vi "Teleop.vi"(10 "Match Info":T1={"Autonomous Elapsed Seconds"=0.0, "TeleOp Elapsed Seconds"=0.0, "Disabled Elapsed Seconds"=0.0, "Visited Autonomous"=FALSE, "Visited TeleOp"=FALSE, "Visited Disabled"=FALSE, "Autonomous Settings"={"Autonomous Style"=enum."Independent", "VI Refnum"=refnum}}, 11 "Call Context":T2) -> ()   [LabVIEW 2017]
doc: "This VI is called for each TeleOp packet received from the DS where the robot is not disabled. It is often used to read from the joysticks and update I/O or to update setpoints for timed control loops. It should complete and return within 20 milliseconds or it may miss DS packets."
uses:
  <vilib>/Rock Robotics/WPI/DriverStation/WPI_DriverStationDerivedRobotMode.ctl
  <vilib>/Rock Robotics/WPI/DriverStation/WPI_DriverStationMatch Info.ctl
  <vilib>/Rock Robotics/WPI/ThirdParty/Phoenix-LabVIEW/Motor Controller/Controls/CTRE_Phoenix_MotorControl_ControlMode.ctl
  <vilib>/Rock Robotics/WPI/Solenoid/WPI_SolenoidValue.ctl
  SCV-Intake2018-master/Change Detect.vi
  SCV-Intake2018-master/Change Detect Boolean.vi
  <vilib>/Rock Robotics/WPI/Utilities/WPI_GetSetVariantRefNum.vi
  <vilib>/Rock Robotics/WPI/Solenoid/WPI_SolenoidSetEnum.vi
panel:
  in  "negInertiaScalar":dbl=0.8
  in  "Sensitivty":dbl=1.15
  in  "WheelNonLinearity":dbl=0.65
  in  "Velocidade constante":dbl=-0.3 format="%#_13g"
  out "Voltage":dbl
  in  "Velocidade Repelir":dbl=0.8
  in  "Velocidade Coletar":dbl=-0.8
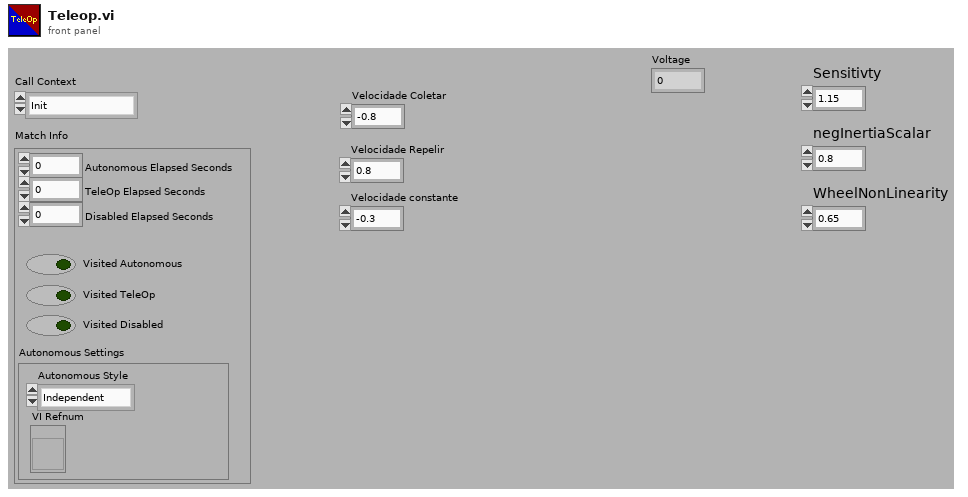
[diagram p1: front panel]
types:
  T1 = typedef "WPI_DriverStationMatch Info.ctl" = cluster{"Autonomous Elapsed Seconds":dbl, "TeleOp Elapsed Seconds":dbl, "Disabled Elapsed Seconds":dbl, "Visited Autonomous":bool, "Visited TeleOp":bool, "Visited Disabled":bool, "Autonomous Settings":cluster{"Autonomous Style":enum16{"Iterative", "Independent"}, "VI Refnum":refnum<vi>}}
  T2 = typedef "WPI_DriverStationDerivedRobotMode.ctl" = enum16{"Init", "Execute", "Stop"}
  T3 = typedef "WPI_SolenoidValue.ctl" = enum16{"Off", "On", "Forward", "Reverse"}
  T4 = typedef "CTRE_Phoenix_MotorControl_ControlMode.ctl" = u16
  T5 = typedef "WPI_AnalogChannelDevRef.ctl" = cluster{"DevStatus":errorcluster, "Analog Channel":T6}
  T6 = typedef "FPGA_AIChannel.ctl" = enum8{"AI 0", "AI 1", "AI 2", "AI 3", "AI MXP 0", "AI MXP 1", "AI MXP 2", "AI MXP 3", "Invalid"}
  T7 = typedef "WPI_JoystickDevRef.ctl" = cluster{"Device":T8}
  T8 = typedef "WPI_JoystickDeviceEnum.ctl" = enum16{"USB 0", "USB 1", "USB 2", "USB 3", "USB 4", "USB 5"}
  T9 = cluster{"Axes[0]":dbl, "Axes[1]":dbl, "Axes[2]":dbl, "Axes[3]":dbl, "Axes[4]":dbl, "Axes[5]":dbl, "Axes[6]":dbl, "Axes[7]":dbl, "Axes[8]":dbl}
  T10 = cluster{"Buttons[0]":bool, "Buttons[1]":bool, "Buttons[2]":bool, "Buttons[3]":bool, "Buttons[4]":bool, "Buttons[5]":bool, "Buttons[6]":bool, "Buttons[7]":bool, "Buttons[8]":bool}
  T11 = typedef "WPI_MotorControlDeviceRef.ctl" = cluster{"DeviceStatus":errorcluster, "Type":T12, "PWM":cluster{"PWM Channel":T13, "DeadBand":T14}, "CAN":cluster{"Device Number":u8, "SetOutput VI Ref":variant, "GetOutput VI Ref":variant, "Enable VI Ref":variant, "Disable VI Ref":variant, "Data":variant}, "Invert":bool, "DIO PWM":cluster{"PWM \"Enable\" Channel":T13, "DIOChannel":T15, "PWM Rate":dbl}}
  T12 = typedef "WPI_MotorControlType.ctl" = enum16{"PWM", "CAN", "DIO PWM"}
  T13 = typedef "FPGA_DIOPWMChannel.ctl" = enum8{"PWM 0", "PWM 1", "PWM 2", "PWM 3", "PWM 4", "PWM 5", "PWM 6", "PWM 7", "PWM 8", "PWM 9", "PWM MXP 0", "PWM MXP 1", "PWM MXP 2", "PWM MXP 3", "PWM MXP 4", "PWM MXP 5", "PWM MXP 6", "PWM MXP 7", "PWM MXP 8", "PWM MXP 9", "Invalid"}
  T14 = typedef "WPI_PWMDeadband.ctl" = cluster{"Name":string, "maxPositivePwm":i32, "minPositivePwm":i32, "centerPwm":i32, "maxNegativePwm":i32, "minNegativePwm":i32, "angularRange":u16}
  T15 = typedef "FPGA_DIOChannel.ctl" = enum8{"DIO 0", "DIO 1", "DIO 2", "DIO 3", "DIO 4", "DIO 5", "DIO 6", "DIO 7", "DIO 8", "DIO 9", "DIO MXP 0", "DIO MXP 1", "DIO MXP 2", "DIO MXP 3", "DIO MXP 4", "DIO MXP 5", "DIO MXP 6", "DIO MXP 7", "DIO MXP 8", "DIO MXP 9", "DIO MXP 10", "DIO MXP 11", "DIO MXP 12", "DIO MXP 13", "DIO MXP 14", "DIO MXP 15", "SPI Port CS1", "SPI Port CS2", "SPI Port CS3", "SPI Port MISO", "SPI Port MOSI", "Invalid"}
  T16 = typedef "WPI_SolenoidDevRef.ctl" = cluster{"DevStatus":errorcluster, "Pneumatics Control Module":u8, "Forward Solenoid Channel":T17, "Reverse Solenoid Channel":T17}
  T17 = typedef "WPI_SolenoidChannel.ctl" = enum8{"Solenoid 0", "Solenoid 1", "Solenoid 2", "Solenoid 3", "Solenoid 4", "Solenoid 5", "Solenoid 6", "Solenoid 7", "Invalid"}
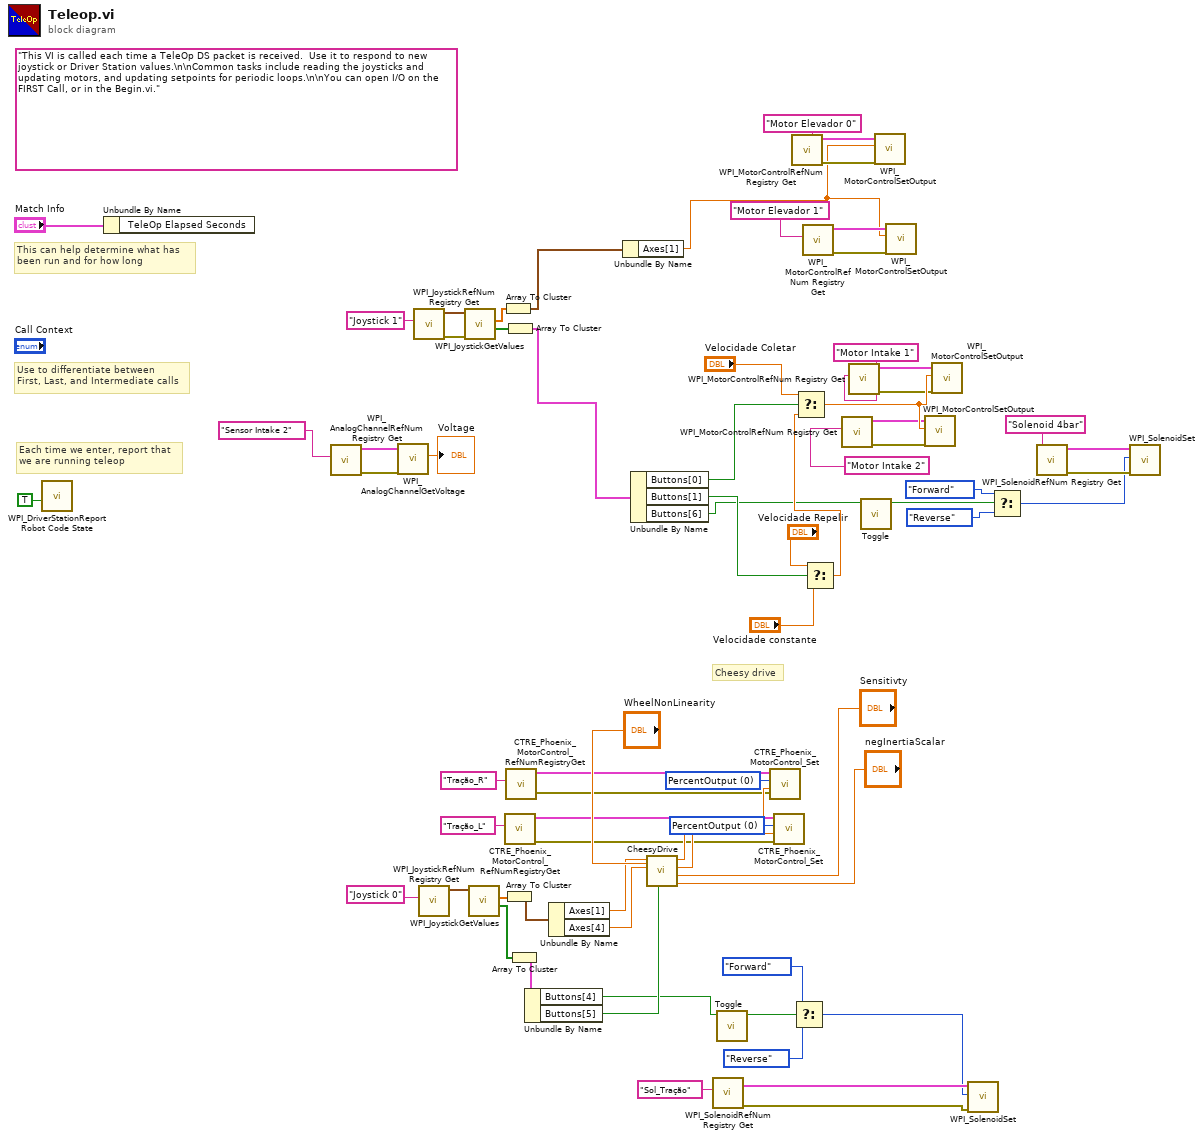
[diagram p0: block diagram]
diagram:
  w18 = T4 0 items=["PercentOutput"=0, "Position"=1, "Velocity"=2, "Current"=3, "Follower"=5, "MotionProfile"=6, "MotionMagic"=7, "MotionMagicArc"=8, "MotionProfileArc"=10, "Disabled"=15] ("Control Mode")
  w19 = T4 0 items=["PercentOutput"=0, "Position"=1, "Velocity"=2, "Current"=3, "Follower"=5, "MotionProfile"=6, "MotionMagic"=7, "MotionMagicArc"=8, "MotionProfileArc"=10, "Disabled"=15] ("Control Mode")
  (unwired) "This VI is called each time a TeleOp DS packet is received.  Use it to respond to new joystick or Driver Station values.\n\nCommon tasks include reading the joysticks and updating motors, and updating setpoints for periodic loops.\n\nYou can open I/O on the FIRST Call, or in the Begin.vi."
  # "Cheesy drive"
  # "Each time we enter, report that\nwe are running teleop"
  # "Use to differentiate between\nFirst, Last, and Intermediate calls"
  # "This can help determine what has\nbeen run and for how long"
  n1 = call <vilib>:"WPI_DriverStationReport Robot Code State.vi"("TeleOp"=TRUE ("Autonomous")) -> ()  [unwired: 10 in, 1 out]
  n2 = Unbundle By Name("Match Info") -> ()  [unwired: 1 out]
  n3 = call <vilib>:"WPI_AnalogChannelRefNum Registry Get.vi"("refnum name"="Sensor Intake 2") -> ("error out"=w64:errorcluster, "AIDeviceRef"=w65:T5)  [unwired: 9 in]
  n4 = call <vilib>:"WPI_AnalogChannelGetVoltage.vi"("error in (no error)"=w64, "AIDeviceRef"=w65) -> ("Voltage"=→"Voltage":dbl)  [unwired: 7 in, 2 out]
  n5 = call <vilib>:"WPI_JoystickRefNum Registry Get.vi"("refnum name"="Joystick 1") -> ("error out"=w69:errorcluster, "JoystickDevRef"=w68:T7)  [unwired: 9 in]
  n6 = call <vilib>:"WPI_JoystickRefNum Registry Get.vi"("refnum name"="Joystick 0") -> ("JoystickDevRef"=w46:T7)  [unwired: 1 in, 9 out]
  n7 = call <vilib>:"WPI_JoystickGetValues.vi"("error in (no error)"=w69, "JoystickDevRef"=w68) -> ("Buttons"=w67:bool[], "Axes"=w9:dbl[])  [unwired: 5 in, 3 out]
  n8 = call <vilib>:"WPI_JoystickGetValues.vi"("JoystickDevRef"=w46) -> ("Buttons"=w41:bool[], "Axes"=w45:dbl[])  [unwired: 6 in, 3 out]
  n9 = Array To Cluster(array=w9) -> (cluster=w8:T9)
  n10 = Array To Cluster(array=w45) -> (cluster=w44:T9)
  n11 = Array To Cluster(array=w67) -> (cluster=w48:T10)
  n12 = call <vilib>:"CTRE_Phoenix_MotorControl_RefNumRegistryGet.vi"("refnum name"="Tração_L") -> ("error out"=w21:errorcluster, "PhoenixMotorControlDevRef"=w22:T11)  [unwired: 9 in]
  n13 = call <vilib>:"CTRE_Phoenix_MotorControl_RefNumRegistryGet.vi"("refnum name"="Tração_R") -> ("error out"=w20:errorcluster, "PhoenixMotorControlDevRef"=w23:T11)  [unwired: 9 in]
  n14 = Array To Cluster(array=w41) -> (cluster=w42:T10)
  n15 = Unbundle By Name(w42) -> ("Buttons[4]"=w28:bool, "Buttons[5]"=w30:bool)
  n16 = Unbundle By Name(w44) -> ("Axes[1]"=w40:dbl, "Axes[4]"=w39:dbl)
  n17 = Unbundle By Name(w8) -> ("Axes[1]"=w3:dbl)
  n18 = Unbundle By Name(w48) -> ("Buttons[0]"=w54:bool, "Buttons[1]"=w60:bool, "Buttons[6]"=w10:bool)
  n19 = call "CheesyDrive.vi"("Quickturn"=w30, "WheelNonLinearity"="WheelNonLinearity", "negInertiaScalar"="negInertiaScalar", "Sensitivty"="Sensitivty", "Wheel"=w39, "Throttle"=w40) -> ("Right PWM"=w25:dbl, "Left PWM"=w24:dbl)  [unwired: 4 in]
  n20 = call <vilib>:"WPI_SolenoidRefNum Registry Get.vi"("refnum name"="Sol_Tração") -> ("error out"=w34:errorcluster, "SolenoidDevRef"=w35:T16)  [unwired: 9 in]
  n21 = call "Toggle.vi"("In"=w28) -> ("Toggled"=w29:bool)  [unwired: 10 in]
  n22 = call <vilib>:"CTRE_Phoenix_MotorControl_Set.vi"("error in (no error)"=w20, "Output"=w24, "Control Mode"=w19, "PhoenixMotorControlDevRef"=w23) -> ()  [unwired: 6 in, 2 out]
  n23 = call <vilib>:"CTRE_Phoenix_MotorControl_Set.vi"("error in (no error)"=w21, "Output"=w25, "Control Mode"=w18, "PhoenixMotorControlDevRef"=w22) -> ()  [unwired: 6 in, 2 out]
  n24 = call <vilib>:"WPI_MotorControlRefNum Registry Get.vi"("refnum name"="Motor Elevador 0") -> ("error out"=w5:errorcluster, "MotorControlDevRef"=w4:T11)  [unwired: 9 in]
  n25 = Select(t=WPI_SolenoidValue."Forward" ("Value"), s=w29, f=WPI_SolenoidValue."Reverse" ("Value")) -> (s? t:f=w31:T3)
  n26 = call <vilib>:"WPI_MotorControlRefNum Registry Get.vi"("refnum name"="Motor Elevador 1") -> ("error out"=w6:errorcluster, "MotorControlDevRef"=w7:T11)  [unwired: 9 in]
  n27 = Select(t="Velocidade Repelir", s=w60, f="Velocidade constante") -> (s? t:f=w61:dbl)
  n28 = Select(t="Velocidade Coletar", s=w54, f=w61) -> (s? t:f=w58:dbl)
  n29 = call <vilib>:"WPI_MotorControlRefNum Registry Get.vi"("refnum name"="Motor Intake 2") -> ("error out"=w56:errorcluster, "MotorControlDevRef"=w55:T11)  [unwired: 9 in]
  n30 = call <vilib>:"WPI_MotorControlRefNum Registry Get.vi"("refnum name"="Motor Intake 1") -> ("error out"=w53:errorcluster, "MotorControlDevRef"=w52:T11)  [unwired: 9 in]
  n31 = call "Toggle.vi"("In"=w10) -> ("Toggled"=w11:bool)  [unwired: 10 in]
  n32 = call <vilib>:"WPI_MotorControlSetOutput.vi"("error in (no error)"=w5, "Output"=w3, "MotorControlDevRef"=w4) -> ()  [unwired: 6 in, 3 out]
  n33 = call <vilib>:"WPI_MotorControlSetOutput.vi"("error in (no error)"=w6, "Output"=w3, "MotorControlDevRef"=w7) -> ()  [unwired: 6 in, 3 out]
  n34 = call <vilib>:"WPI_MotorControlSetOutput.vi"("error in (no error)"=w56, "Output"=w58, "MotorControlDevRef"=w55) -> ()  [unwired: 6 in, 3 out]
  n35 = call <vilib>:"WPI_MotorControlSetOutput.vi"("error in (no error)"=w53, "Output"=w58, "MotorControlDevRef"=w52) -> ()  [unwired: 6 in, 3 out]
  n36 = call-poly <vilib>:"WPI_SolenoidSet.vi"("error in (no error)"=w34, "Value"=w31, "SolenoidDevRef"=w35) -> ()  [unwired: 7 in, 2 out]
  n37 = Select(t=WPI_SolenoidValue."Forward" ("Value"), s=w11, f=WPI_SolenoidValue."Reverse" ("Value")) -> (s? t:f=w14:T3)
  n38 = call <vilib>:"WPI_SolenoidRefNum Registry Get.vi"("refnum name"="Solenoid 4bar") -> ("error out"=w17:errorcluster, "SolenoidDevRef"=w16:T16)  [unwired: 9 in]
  n39 = call-poly <vilib>:"WPI_SolenoidSet.vi"("error in (no error)"=w17, "Value"=w14, "SolenoidDevRef"=w16) -> ()  [unwired: 7 in, 2 out]
